vi "Camera.vi"() -> ()   [LabVIEW 2016]
uses:
  <vilib>/rvi/Emulation/niFpgaGetClockAttributes.vi
  <vilib>/rvi/Emulation/niFpgaSctlEmulationGetInTimedLoop.vi
  <vilib>/rvi/Emulation/niFpgaEmulationReportErrorSimple.vi
  <vilib>/rvi/eio/common/nirviEmuTemplateMethod_errors.vi
  <vilib>/rvi/Emulation/niFpgaCriticalErrorInLSC.vi
  <vilib>/eio/EIONode/EIONode.xnode
panel:
  in  "Tlow = t":i16=9
  in  "Fly View Frame Rate = R":i16=10
  in  "Arena View Frame Rate = R":i16=100
  out "Camera flash time":i16
  in  "Camera flash time t":i16
  in  "Flash":bool
  # "** Frequency  = 1 / (Fly View R * 0.0001)   i.e R = 10, Frequency = 1000Hz"
  # "**T period = R*100µs,      T low = t*100 µs"
  # "** Frequency  = 1 / (R * 0.0001)   i.e R = 100, Frequency = 100Hz"
  # "** Trigger the fluorenscence camera (Arena View R - x ) *100 microseconds earlier\n      i.e Arena View R = 100, x = 98,\n           offset x = (100 - 98) * 100 µs = 200 µs"
  # "** Camera flash time is set to be the time for triggering the flash at the end of every video.\n** The unit is second."
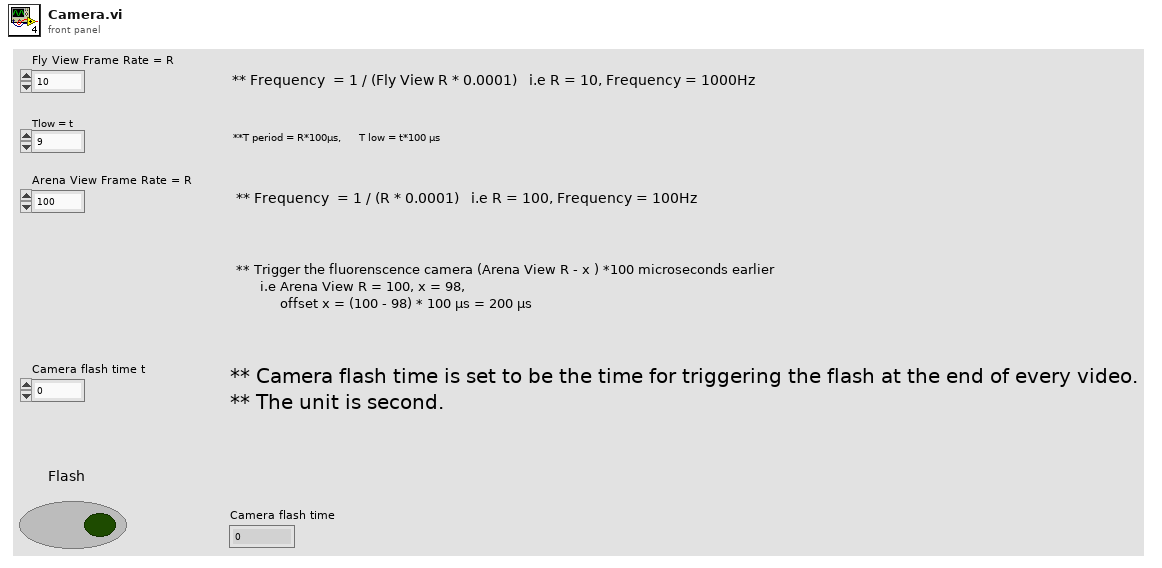
[diagram p1: front panel]
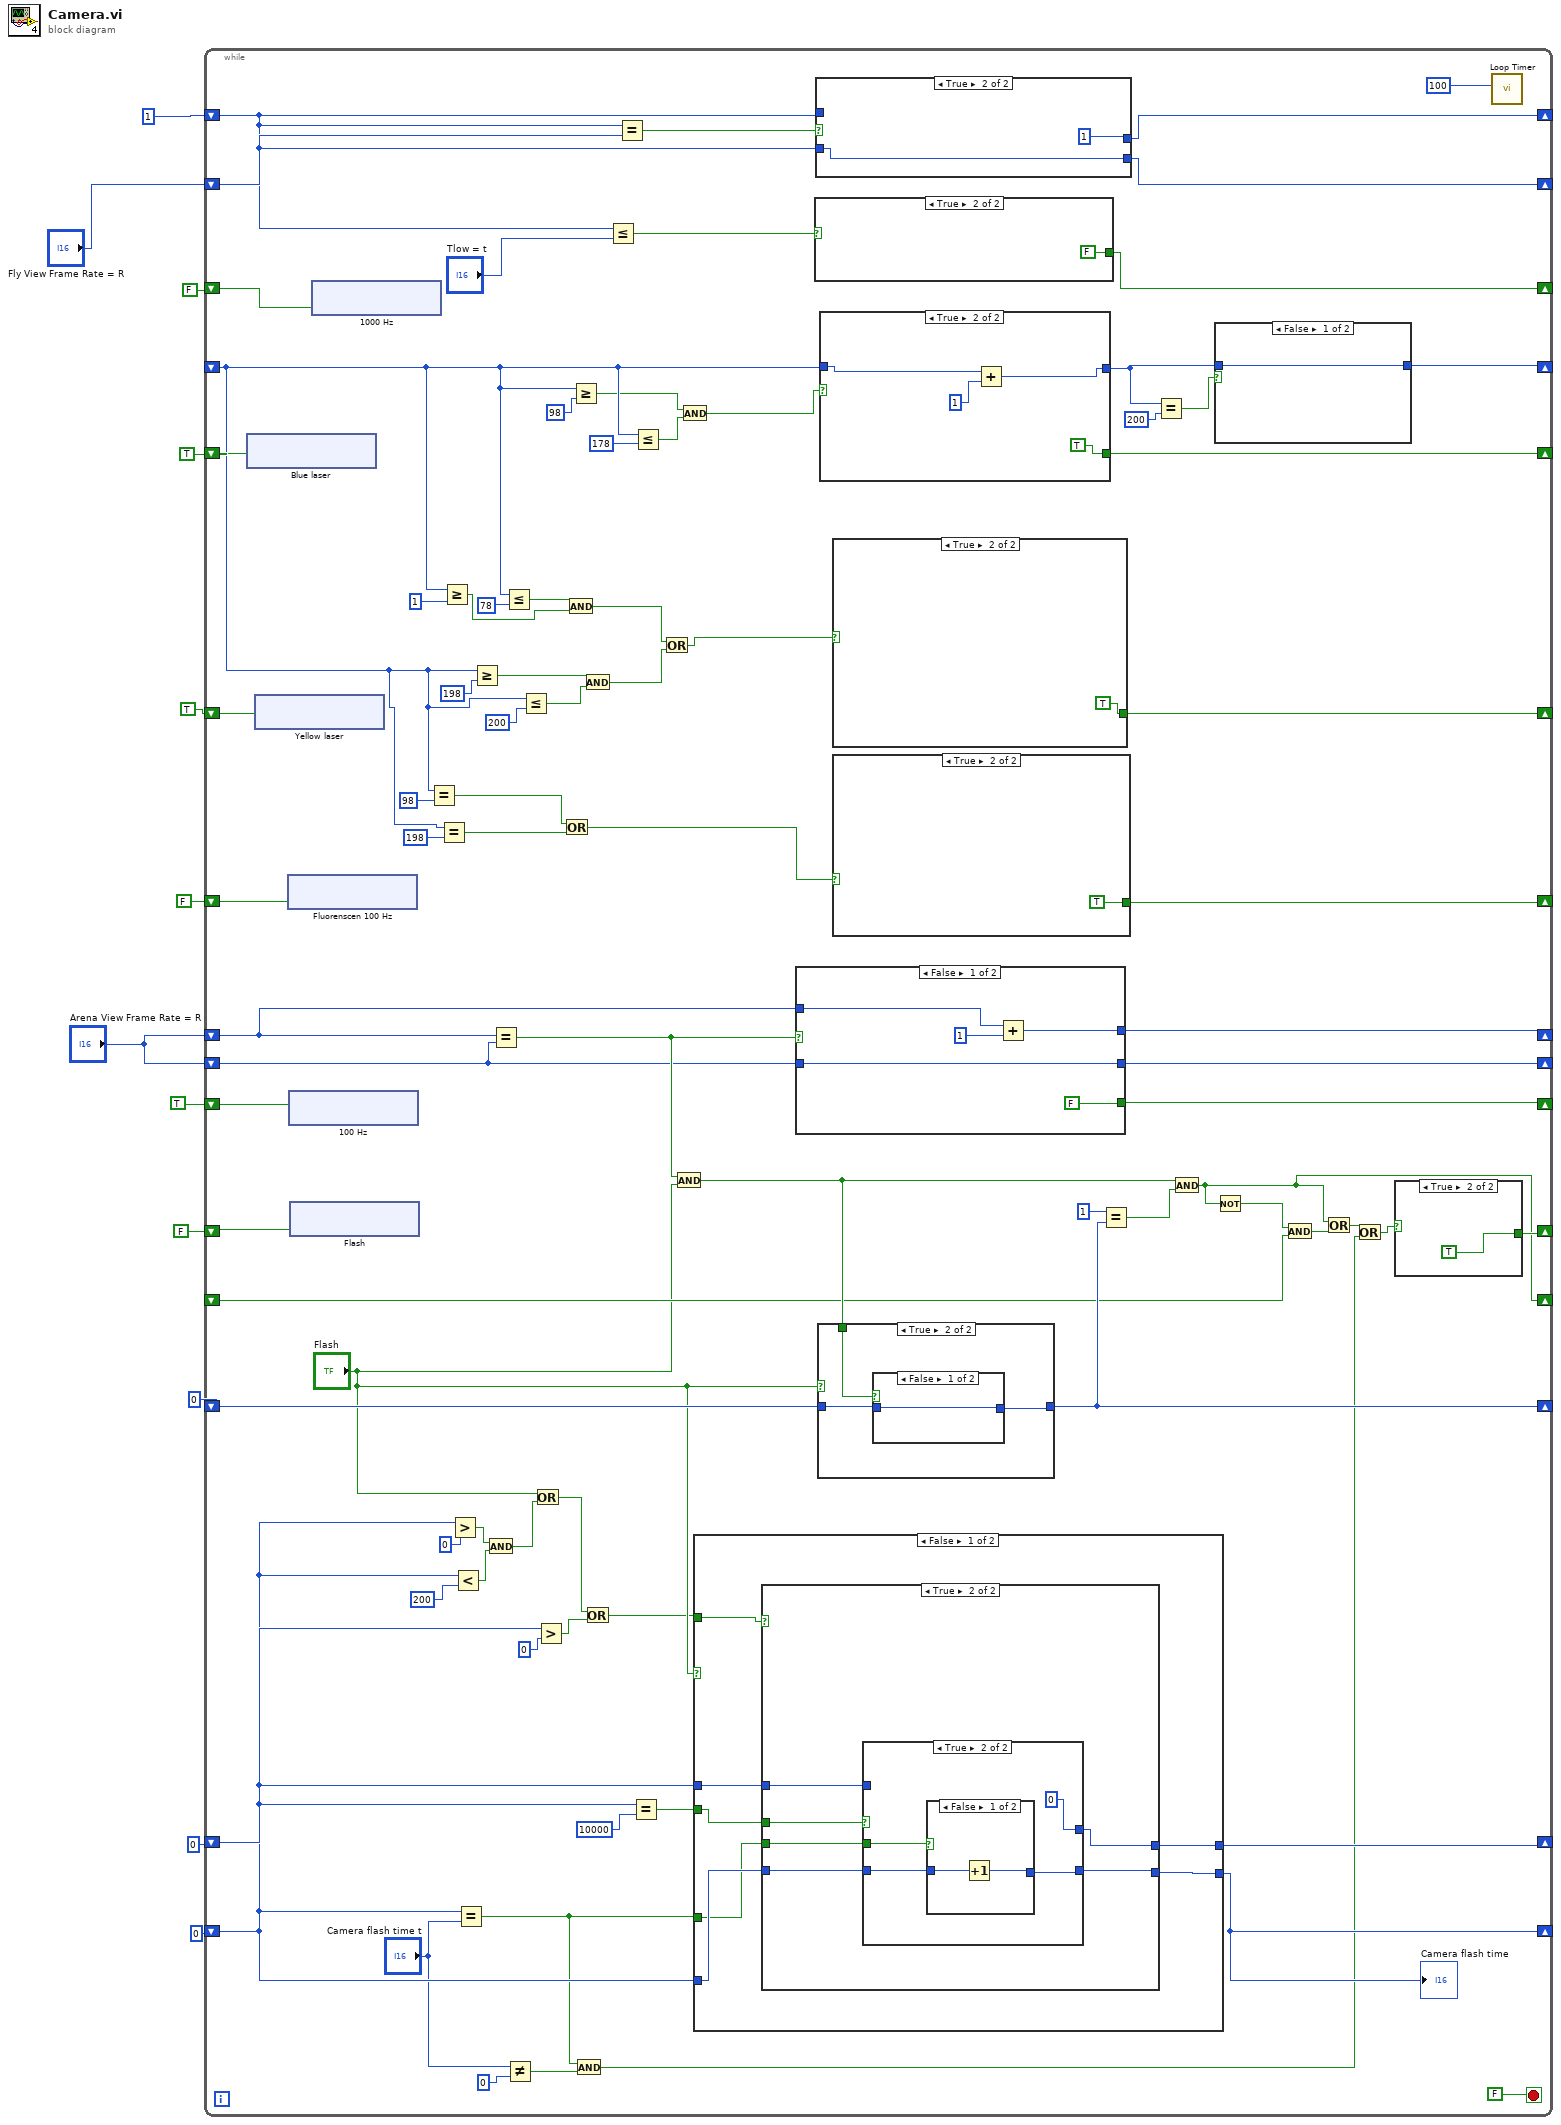
[diagram p0: block diagram]
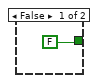
[diagram p2: hidden frame]
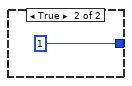
[diagram p3: hidden frame]
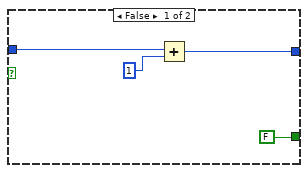
[diagram p4: hidden frame]
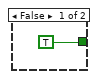
[diagram p5: hidden frame]
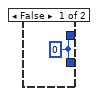
[diagram p6: hidden frame]
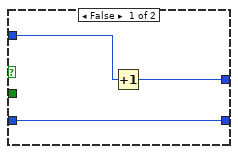
[diagram p7: hidden frame]
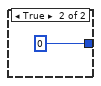
[diagram p8: hidden frame]
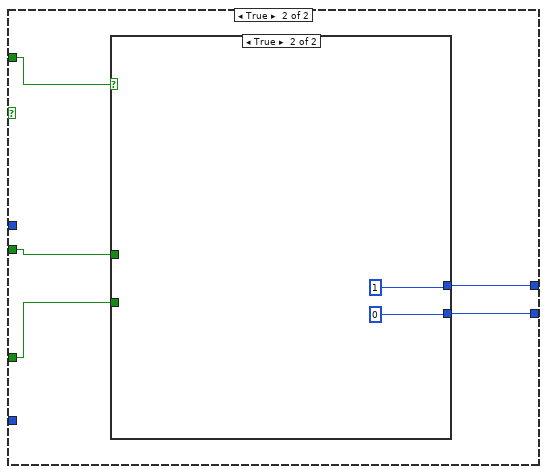
[diagram p9: hidden frame]
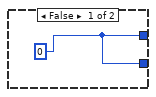
[diagram p10: hidden frame]
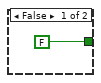
[diagram p11: hidden frame]
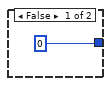
[diagram p12: hidden frame]
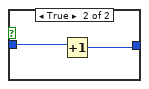
[diagram p13: hidden frame]
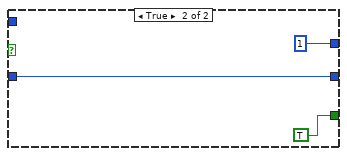
[diagram p14: hidden frame]
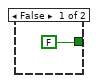
[diagram p15: hidden frame]
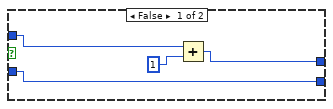
[diagram p16: hidden frame]
diagram:
  n1 = while {
    shift-right: [w47] -> _
    shift-left: FALSE -> [w96]
    shift-right: [w94] -> _
    shift-left: i16 1 -> [w43]
    shift-right: [w92] -> _
    shift-left: FALSE -> [w93]
    shift-right: [w91] -> _
    shift-left: TRUE -> [w86]
    shift-right: [w90] -> _
    shift-left: "Arena View Frame Rate = R" -> [w81]
    shift-right: [w83] -> _
    shift-left: i16 0 -> [w87]
    shift-right: [w79] -> _
    shift-left: FALSE -> [w80]
    shift-right: [w75] -> _
    shift-left: _ -> [w76]
    shift-right: [w69] -> _
    shift-left: i16 0 -> [w62]
    shift-right: [w70] -> _
    shift-left: i16 0 -> [w56]
    shift-right: [w50] -> _
    shift-left: "Arena View Frame Rate = R" -> [w49]
    shift-right: [w48] -> _
    shift-left: "Fly View Frame Rate = R" -> [w46]
    shift-right: [w38] -> _
    shift-left: _ -> [w16]
    shift-right: [w41] -> _
    shift-left: TRUE -> [w42]
    shift-right: [w35] -> _
    shift-left: TRUE -> [w36]
    stop <- FALSE stop-if-true
    n2 = xnode "Blue laser"("ConnectorC/DIO4"=w42) -> ()  [unwired: 1 in, 1 out]
    n3 = xnode "Yellow laser"("ConnectorC/DIO5"=w36) -> ()  [unwired: 1 in, 1 out]
    n4 = xnode "Fluorenscen 100 Hz"("ConnectorC/DIO1"=w93) -> ()  [unwired: 1 in, 1 out]
    n5 = xnode "100 Hz"("ConnectorC/DIO2"=w86) -> ()  [unwired: 1 in, 1 out]
    n6 = xnode "Flash"("ConnectorC/DIO3"=w80) -> ()  [unwired: 1 in, 1 out]
    n7 = xnode "1000 Hz"("ConnectorC/DIO0"=w96) -> ()  [unwired: 1 in, 1 out]
    n8 = Equal?(x=w16, y=i16 98) -> (x = y?=w33:bool)
    n9 = Equal?(x=w16, y=i16 198) -> (x = y?=w31:bool)
    n10 = Greater Or Equal?(x=w16, y=i16 1) -> (x >= y?=w20:bool)
    n11 = Greater?(x=w56, y=i16 0) -> (0:w59:bool)
    n12 = Less?(x=w56, y=i16 200) -> (x < y?=w58:bool)
    n13 = Equal?(x=w56, y="Camera flash time t") -> (x = y?=w52:bool)
    n14 = Greater Or Equal?(x=w16, y=i16 198) -> (x >= y?=w23:bool)
    n15 = And(x=w59, y=w58) -> (x .and. y?=w57:bool)
    n16 = Equal?(x=w81, y=w49) -> (x = y?=w88:bool)
    n17 = Less Or Equal?(x=w16, y=i16 78) -> (x <= y?=w21:bool)
    n18 = Not Equal?(x="Camera flash time t", y=i16 0) -> (x != y?=w53:bool)
    n19 = Less Or Equal?(x=w16, y=i16 200) -> (x <= y?=w24:bool)
    n20 = Or(x="Flash", y=w57) -> (x .or. y?=w64:bool)
    n21 = Greater?(x=w62, y=i16 0) -> (0:w65:bool)
    n22 = Or(x=w33, y=w31) -> (x .or. y?=w30:bool)
    n23 = And(x=w21, y=w20) -> (x .and. y?=w19:bool)
    n24 = Greater Or Equal?(x=w16, y=i16 98) -> (x >= y?=w15:bool)
    n25 = And(x=w52, y=w53) -> (x .and. y?=w51:bool)
    n26 = And(x=w23, y=w24) -> (x .and. y?=w22:bool)
    n27 = Or(x=w64, y=w65) -> (x .or. y?=w63:bool)
    n28 = Less Or Equal?(x=w43, y="Tlow = t") -> (x <= y?=w45:bool)
    n29 = Equal?(x=w43, y=w46) -> (x = y?=w89:bool)
    n30 = Equal?(x=w62, y=i16 10000) -> (x = y?=w68:bool)
    n31 = Less Or Equal?(x=w16, y=i16 178) -> (x <= y?=w14:bool)
    n32 = Or(x=w19, y=w22) -> (x .or. y?=w29:bool)
    n33 = And(x=w88, y="Flash") -> (x .and. y?=w85:bool)
    n34 = And(x=w15, y=w14) -> (x .and. y?=w13:bool)
    n35 = case shown="False" "Flash" {
      tunnel: [w116 w139] -> w70
      tunnel: [w117 w138] -> w69
      tunnel: w62 -> [w114 _]
      tunnel: w68 -> [w115 w137]
      tunnel: w52 -> [w111 w136]
      tunnel: w56 -> [w113 _]
      tunnel: w63 -> [w112 w135]
      frame False {
        n36 = case shown="True" w112 {
          tunnel: [w118 w122] -> w117
          tunnel: [w118 w121] -> w116
          tunnel: w115 -> [_ w124]
          tunnel: w114 -> [_ w123]
          tunnel: w113 -> [_ w120]
          tunnel: w111 -> [_ w119]
          frame False {
            w118 = i16 0
          }
          frame True {
            n37 = case shown="True" w124 {
              tunnel: w123 -> [w127 _]
              tunnel: [w126 i16 0] -> w122
              tunnel: [w125 w130] -> w121
              tunnel: w120 -> [w125 w129]
              tunnel: w119 -> [_ w128]
              frame False {
                n38 = Increment(x=w127) -> (x+1=w126:i16)
              }
              frame True {
                n39 = case shown="False" w128 {
                  tunnel: [w132 i16 0] -> w130
                  tunnel: w129 -> [w133 _]
                  frame False {
                    n40 = Increment(x=w133) -> (x+1=w132:i16)
                  }
                  frame True {
                  }
                }
              }
            }
          }
        }
      }
      frame True {
        n41 = case shown="True" w135 {
          tunnel: [w140 i16 1] -> w138
          tunnel: w136 -> [_ _]
          tunnel: [w140 i16 0] -> w139
          tunnel: w137 -> [_ _]
          frame False {
            w140 = i16 0
          }
          frame True {
          }
        }
      }
    }
    "Camera flash time" <- w70
    n42 = case shown="False" w88 {
      tunnel: [FALSE TRUE] -> w91
      tunnel: [w154 i16 1] -> w90
      tunnel: w81 -> [w156 _]
      tunnel: [w152 w157] -> w50
      tunnel: w49 -> [w152 w157]
      frame False {
        n43 = Add(x=w156, y=i16 1) -> (x+y=w154:i16)
      }
      frame True {
      }
    }
    n44 = case shown="True" w45 {
      tunnel: [TRUE FALSE] -> w47
      frame False {
      }
      frame True {
      }
    }
    n45 = case shown="True" w89 {
      tunnel: [w164 i16 1] -> w94
      tunnel: w43 -> [w163 _]
      tunnel: [w162 w166] -> w48
      tunnel: w46 -> [w162 w166]
      frame False {
        n46 = Add(x=w163, y=i16 1) -> (x+y=w164:i16)
      }
      frame True {
      }
    }
    n47 = case shown="True" "Flash" {
      tunnel: w87 -> [_ w147]
      tunnel: [i16 0 w146] -> w83
      tunnel: w85 -> [_ w148]
      frame False {
      }
      frame True {
        n48 = case shown="False" w148 {
          tunnel: w147 -> [w149 w151]
          tunnel: [w149 w150] -> w146
          frame False {
          }
          frame True {
            n49 = Increment(x=w151) -> (x+1=w150:i16)
          }
        }
      }
    }
    n50 = case shown="True" w13 {
      tunnel: w16 -> [w103 w106]
      tunnel: [w102 w105] -> w37
      tunnel: [FALSE TRUE] -> w41
      frame False {
        n51 = Add(x=w103, y=i16 1) -> (x+y=w102:i16)
      }
      frame True {
        n52 = Add(x=w106, y=i16 1) -> (x+y=w105:i16)
      }
    }
    n53 = case shown="True" w29 {
      tunnel: [FALSE TRUE] -> w35
      frame False {
      }
      frame True {
      }
    }
    n54 = case shown="True" w30 {
      tunnel: [FALSE TRUE] -> w92
      frame False {
      }
      frame True {
      }
    }
    n55 = Equal?(x=i16 1, y=w83) -> (x = y?=w82:bool)
    n56 = Equal?(x=w37, y=i16 200) -> (x = y?=w39:bool)
    n57 = And(x=w85, y=w82) -> (x .and. y?=w75:bool)
    n58 = case shown="False" w39 {
      tunnel: [w99 i16 1] -> w38
      tunnel: w37 -> [w99 _]
      frame False {
      }
      frame True {
      }
    }
    n59 = Not(x=w75) -> (.not. x?=w77:bool)
    n60 = And(x=w77, y=w76) -> (x .and. y?=w78:bool)
    n61 = Or(x=w75, y=w78) -> (x .or. y?=w73:bool)
    n62 = Or(x=w73, y=w51) -> (x .or. y?=w72:bool)
    n63 = case shown="True" w72 {
      tunnel: [FALSE TRUE] -> w79
      frame False {
      }
      frame True {
      }
    }
    n64 = call "Loop Timer"("Count(uSec)"=u32 100) -> ()  [unwired: 1 out]
  }
